vi "PING))) demo(not).vi"() -> ()   [LabVIEW 2016]
uses:
  <vilib>/myRIO/Instrument Drivers/Onboard IO/DIO/typedefs/DIO Reference.ctl
  <vilib>/myRIO/Common/Instrument Driver Framework/Utilities/typedefs/myRIO Generic Hardware Reference.ctl
  <vilib>/myRIO/Common/Instrument Driver Framework/Utilities/typedefs/Hardware Version Enum.ctl
  <vilib>/myRIO/Common/Instrument Driver Framework/Utilities/typedefs/myRIO v1.0 Reference.ctl
  <vilib>/myRIO/Common/Instrument Driver Framework/Utilities/typedefs/Generic FPGA Reference.ctl
  <vilib>/myRIO/Common/Instrument Driver Framework/myRIO v1.0/DIO/typedefs/DIO Channels List.ctl
  <vilib>/myRIO/Common/Instrument Driver Framework/myRIO v1.0/DIO/typedefs/DIO Channels Enum.ctl
  <vilib>/myRIO/Common/Instrument Driver Framework/myRIO v1.0/DIO/vis/myRIO v1.0 Close DIO.vi
  <vilib>/myRIO/Common/Instrument Driver Framework/myRIO v1.0/DIO/vis/myRIO v1.0 Unreserve DIO.vi
  <vilib>/myRIO/Common/Instrument Driver Framework/myRIO v1.0/DIO/vis/myRIO v1.0 Build MUX Configuration DIO.vi
  <vilib>/myRIO/Common/Instrument Driver Framework/myRIO v1.0/Resource Manager/vis/myRIO v1.0 Unreserve Channel List.vi
  <vilib>/myRIO/Common/Instrument Driver Framework/myRIO v1.0/Resource Manager/vis/myRIO v1.0 Create Configuration List.vi
  <vilib>/myRIO/Common/Instrument Driver Framework/myRIO v1.0/Resource Manager/vis/myRIO v1.0 Unreserve Channel.vi
  <vilib>/myRIO/Common/Instrument Driver Framework/myRIO v1.0/Resource Manager/vis/myRIO v1.0 Build Mutex Name.vi
  <vilib>/Utility/error.llb/Error Cluster From Error Code.vi
  <vilib>/myRIO/Common/Instrument Driver Framework/myRIO v1.0/DIO/vis/myRIO v1.0 Write DIO.vi
  <vilib>/myRIO/Common/Instrument Driver Framework/myRIO v1.0/DIO/vis/myRIO v1.0 Read DIO.vi
  <vilib>/myRIO/Common/Instrument Driver Framework/myRIO v1.0/DIO/vis/myRIO v1.0 Shutdown DIO.vi
  <vilib>/myRIO/Common/Instrument Driver Framework/myRIO v1.0/Resource Manager/vis/myRIO v1.0 Configure IO.vi
  <vilib>/myRIO/Common/Instrument Driver Framework/Utilities/vis/Configuration Manager.vi
  <vilib>/myRIO/Common/Instrument Driver Framework/Utilities/vis/IO Manager.vi
  <vilib>/myRIO/Common/Instrument Driver Framework/myRIO v1.0/myRIO v1.0 Close.vi
  <vilib>/myRIO/Instrument Drivers/Onboard IO/DIO/DIO.lvlib
panel:
  out "distance":u32
  in  "Channel Names":tag[](array[tag])
  out "Enum":T1(ring)
  in  "error in (no error)":errorcluster
  in  "stop":bool
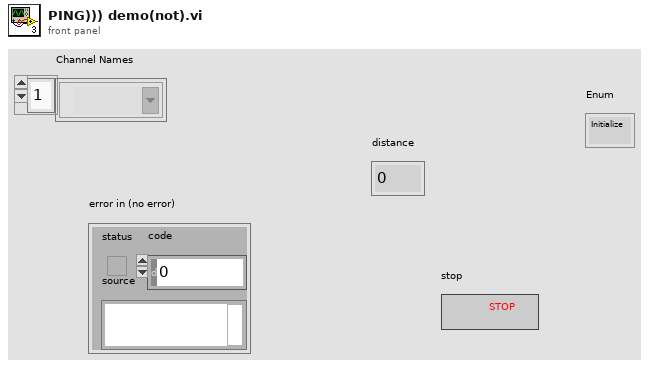
[diagram p1: front panel]
types:
  T1 = enum16{"Initialize", "Trigger pulse", "Wait pulse 1", "Wait pulse 2", "Calculate", "Stop"}
  T2 = typedef "DIO.lvlib/DIO Reference.ctl" = cluster{"myRIO Reference":T3, "DIO Channels List":T7}
  T3 = typedef "myRIO Generic Hardware Reference.ctl" = cluster{"myRIO Model":T4, "myRIO Hardware Reference":T5}
  T4 = typedef "Hardware Version Enum.ctl" = enum16{"Unknown", "myRIO-1900", "myRIO-1950", "roboRIO", "NI ELVIS RIO CM"}
  T5 = typedef "myRIO v1.0 Reference.ctl" = cluster{"Generic FPGA Reference":T6, "Allow multiple opens":bool}
  T6 = typedef "Generic FPGA Reference.ctl" = refnum<k20>
  T7 = typedef "DIO Channels List.ctl" = T8[]
  T8 = typedef "DIO Channels Enum.ctl" = enum16{"Not Connected", "C/DIO0", "C/DIO1", "C/DIO2", "C/DIO3", "C/DIO4", "C/DIO5", "C/DIO6", "C/DIO7", "A/DIO0", "A/DIO1", "A/DIO2", "A/DIO3", "A/DIO4", "A/DIO5", "A/DIO6", "A/DIO7", "A/DIO8", "A/DIO9", "A/DIO10", "A/DIO11", "A/DIO12", "A/DIO13", "A/DIO14", "A/DIO15", "B/DIO0", "B/DIO1", "B/DIO2", "B/DIO3", "B/DIO4", "B/DIO5", "B/DIO6", "B/DIO7", "B/DIO8", "B/DIO9", "B/DIO10", "B/DIO11", "B/DIO12", "B/DIO13", "B/DIO14", "B/DIO15", "LED0", "LED1", "LED2", "LED3", "Button0", "DIO/DIO0", "DIO/DIO1", "DIO/DIO2", "DIO/DIO3", "DIO/DIO4", "DIO/DIO5", "DIO/DIO6", "DIO/DIO7", "DIO/DIO8", "DIO/DIO9", "SPI/CS0", "SPI/CS1", "SPI/CS2", "SPI/CS3", "LED RADIO (Green)", "LED RADIO (Red)", "LED COMM (Green)", "LED COMM (Red)", "LED MODE (Green)", "LED MODE (Red)"}
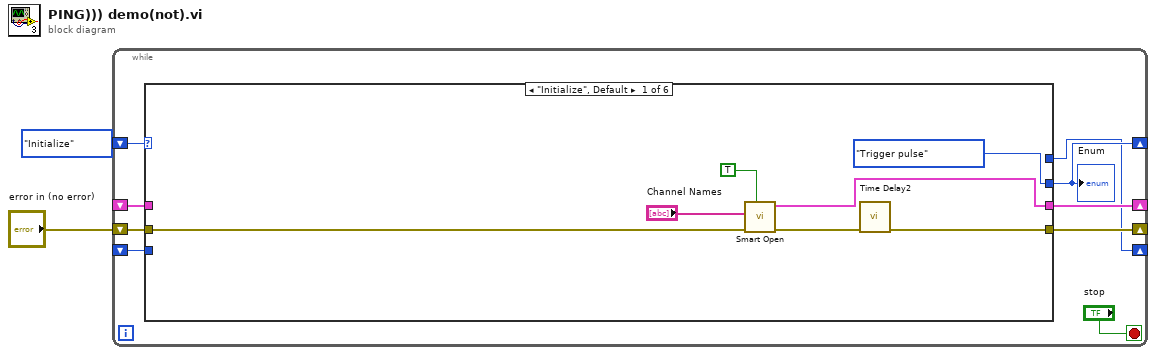
[diagram p0: block diagram]
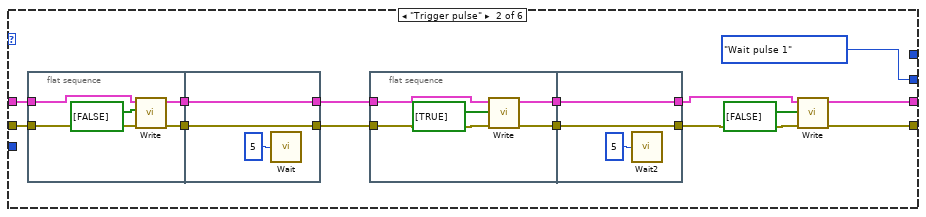
[diagram p2: hidden frame]
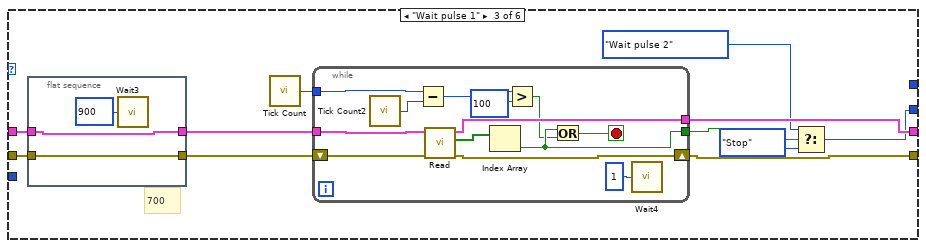
[diagram p3: hidden frame]
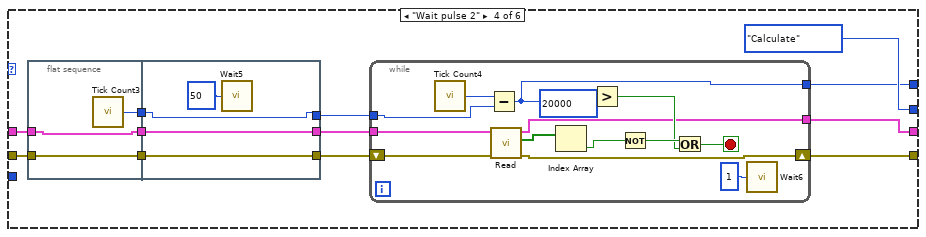
[diagram p4: hidden frame]
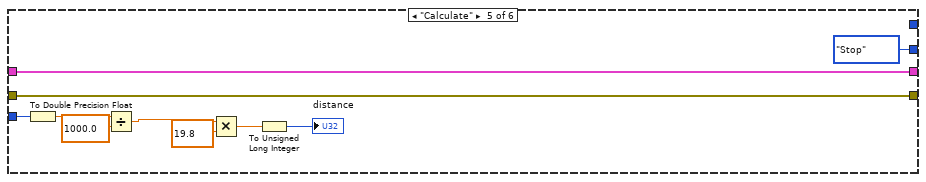
[diagram p5: hidden frame]
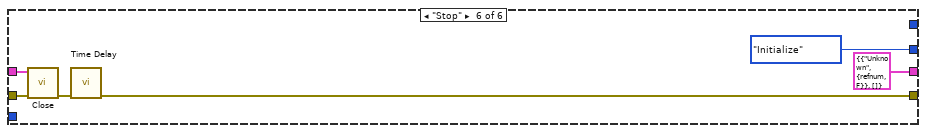
[diagram p6: hidden frame]
diagram:
  n1 = while {
    shift-right: [w9] -> _
    shift-left: T1."Initialize" -> [w10]
    shift-right: [w7] -> _
    shift-left: _ -> [w6]
    shift-right: [w5] -> _
    shift-left: "error in (no error)" -> [w8]
    shift-right: [w3] -> _
    shift-left: _ -> [w4]
    stop <- "stop" stop-if-true
    n2 = case shown="\"Initialize\", Default" w10 {
      tunnel: [T1."Trigger pulse" T1."Wait pulse 1" w50 T1."Calculate" T1."Stop" T1."Initialize"] -> w9
      tunnel: w8 -> [w17 w30 w58 w79 w113 w122]
      tunnel: [w16 w20 w55 w76 w114 T2 {"myRIO Reference"={"myRIO Model"=enum."Unknown", "myRIO Hardware Reference"={"Generic FPGA Reference"=refnum, "Allow multiple opens"=FALSE}}, "DIO Channels List"=[]} ("DIO Ref Out")] -> w7
      tunnel: w6 -> [_ w27 w56 w82 w114 w123]
      tunnel: [w13 w19 w54 w77 w113 w119] -> w5
      tunnel: w4 -> [_ _ _ _ w115 _]
      tunnel: [_ _ _ w78 _ _] -> w3
      frame "Initialize", Default {
        n3 = call <vilib>:"Smart Open.vi"("Allow multiple opens?"=TRUE, "error in (no error)"=w17, "Channel Names"="Channel Names") -> ("error out"=w15:errorcluster, "DIO Ref Out"=w16:T2)  [unwired: 7 in]
        n4 = call "Time Delay2"("error in (no error)"=w15) -> ("error out"=w13:errorcluster)  [unwired: 10 in]
      }
      frame "Trigger pulse" {
        n5 = flat-sequence {
          tunnel: w30 -> [w44]
          tunnel: [w43] -> w28
          tunnel: w27 -> [w42]
          tunnel: [w41] -> w25
          tunnel: [w47] -> w29
          tunnel: w28 -> [w47]
          tunnel: [w46] -> w26
          tunnel: w25 -> [w46]
          frame #0 {
            n6 = call <vilib>:"Write.vi"("error in (no error)"=w44, "Values"=bool[] [FALSE], "DIO Ref In"=w42) -> ("error out"=w43:errorcluster, "DIO Ref Out"=w41:T2)  [unwired: 6 in]
          }
          frame #1 {
            n7 = call "Wait"("Count(uSec)"=u32 5) -> ()  [unwired: 1 out]
          }
        }
        n8 = flat-sequence {
          tunnel: w29 -> [w36]
          tunnel: w26 -> [w35]
          tunnel: [w34] -> w24
          tunnel: [w33] -> w22
          tunnel: w24 -> [w39]
          tunnel: [w39] -> w23
          tunnel: w22 -> [w38]
          tunnel: [w38] -> w21
          frame #0 {
            n9 = call <vilib>:"Write.vi"("error in (no error)"=w36, "Values"=bool[] [TRUE], "DIO Ref In"=w35) -> ("error out"=w33:errorcluster, "DIO Ref Out"=w34:T2)  [unwired: 6 in]
          }
          frame #1 {
            n10 = call "Wait2"("Count(uSec)"=u32 5) -> ()  [unwired: 1 out]
          }
        }
        n11 = call <vilib>:"Write.vi"("error in (no error)"=w21, "Values"=bool[] [FALSE], "DIO Ref In"=w23) -> ("error out"=w19:errorcluster, "DIO Ref Out"=w20:T2)  [unwired: 6 in]
      }
      frame "Wait pulse 1" {
        # "700"
        n12 = flat-sequence {
          tunnel: [w74] -> w59
          tunnel: w58 -> [w74]
          tunnel: [w73] -> w57
          tunnel: w56 -> [w73]
          frame #0 {
            n13 = call "Wait3"("Count(uSec)"=u32 900) -> ()  [unwired: 1 out]
          }
        }
        n14 = call "Tick Count"() -> ("Tick Count(uSec)"=w53:u32)
        n15 = while {
          tunnel: w57 -> [w71]
          tunnel: [w70] -> w55
          shift-right: [w67] -> w54
          shift-left: w59 -> [w72]
          tunnel: w53 -> [w62]
          tunnel: [w61] -> w49
          stop <- w68 stop-if-true
          n16 = call "Tick Count2"() -> ("Tick Count(uSec)"=w63:u32)
          n17 = Subtract(x=w62, y=w63) -> (x-y=w64:u32)
          n18 = call <vilib>:"Read.vi"("error in (no error)"=w72, "DIO Ref In"=w71) -> ("error out"=w67:errorcluster, "Values"=w69:bool[], "DIO Ref Out"=w70:T2)  [unwired: 7 in]
          n19 = Index Array(array=w69) -> (element=w61:bool)  [unwired: 1 in]
          n20 = Greater?(x=w64, y=u32 100) -> (0:w60:bool)
          n21 = Or(x=w61, y=w60) -> (x .or. y?=w68:bool)
          n22 = call "Wait4"("Count(uSec)"=u32 1) -> ()  [unwired: 1 out]
        }
        n23 = Select(t=T1."Wait pulse 2", s=w49, f=T1."Stop") -> (s? t:f=w50:T1)
      }
      frame "Wait pulse 2" {
        n24 = flat-sequence {
          tunnel: [w104] -> w85
          tunnel: [w103] -> w83
          tunnel: w82 -> [w103]
          tunnel: [w102] -> w80
          tunnel: w79 -> [w102]
          tunnel: [w107] -> w86
          tunnel: w85 -> [w107]
          tunnel: [w106] -> w84
          tunnel: w83 -> [w106]
          tunnel: [w105] -> w81
          tunnel: w80 -> [w105]
          frame #0 {
            n25 = call "Tick Count3"() -> ("Tick Count(uSec)"=w104:u32)
          }
          frame #1 {
            n26 = call "Wait5"("Count(uSec)"=u32 50) -> ()  [unwired: 1 out]
          }
        }
        n27 = while {
          tunnel: w86 -> [w89]
          tunnel: w84 -> [w101]
          tunnel: [w93] -> w78
          tunnel: [w90] -> w76
          shift-right: [w91] -> w77
          shift-left: w81 -> [w100]
          stop <- w96 stop-if-true
          n28 = call "Tick Count4"() -> ("Tick Count(uSec)"=w88:u32)
          n29 = Subtract(x=w88, y=w89) -> (x-y=w93:u32)
          n30 = call <vilib>:"Read.vi"("error in (no error)"=w100, "DIO Ref In"=w101) -> ("error out"=w91:errorcluster, "Values"=w99:bool[], "DIO Ref Out"=w90:T2)  [unwired: 7 in]
          n31 = Index Array(array=w99) -> (element=w97:bool)  [unwired: 1 in]
          n32 = Greater?(x=w93, y=u32 20000) -> (0:w95:bool)
          n33 = Not(x=w97) -> (.not. x?=w98:bool)
          n34 = Or(x=w98, y=w95) -> (x .or. y?=w96:bool)
          n35 = call "Wait6"("Count(uSec)"=u32 1) -> ()  [unwired: 1 out]
        }
      }
      frame "Calculate" {
        n36 = To Double Precision Float(number=w115) -> (double precision float=w117:dbl)
        n37 = Divide(x=w117, y=1000.0) -> (x/y=w111:dbl)
        n38 = Multiply(x=w111, y=19.8) -> (x*y=w110:dbl)
        n39 = To Unsigned Long Integer(number=w110) -> (unsigned 32bit integer=→"distance":u32)
      }
      frame "Stop" {
        n40 = call <vilib>:"Close.vi"("error in (no error)"=w122, "DIO Ref In"=w123) -> ("error out"=w120:errorcluster)  [unwired: 9 in]
        n41 = call "Time Delay"("error in (no error)"=w120) -> ("error out"=w119:errorcluster)  [unwired: 10 in]
      }
    }
    "Enum" <- w9
  }
